vi "Host_SaveToFile.vi"() -> ()   [LabVIEW 2017]
doc: "Dialogue window shows user input for file name.\nSaves all data taken to a file in Data folder.\nIf the explore button is pressed instead, the file explorer wiill be openend and will save data to the specified location."
uses:
  <vilib>/Utility/file.llb/Write Delimited Spreadsheet (string).vi
  Globals/Host_DATAALL.vi
panel:
  in  "Flush Data":bool
  in  "Custom Path":bool
  in  "cancel":bool
  in  "OK Button":bool
  in  "File name":string caption="Enter File Name:"
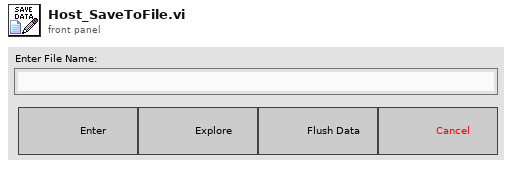
[diagram p1: front panel]
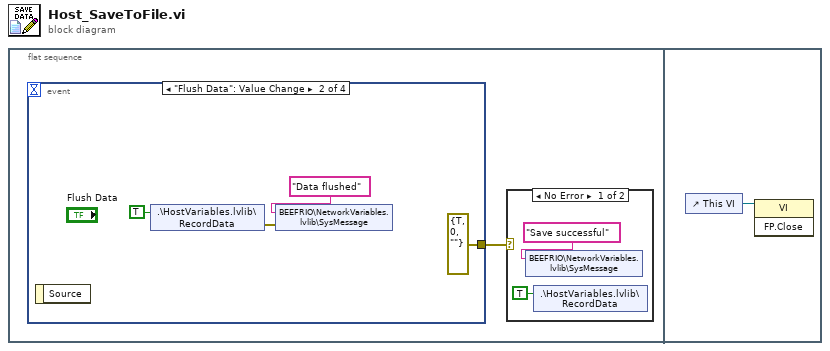
[diagram p0: block diagram]
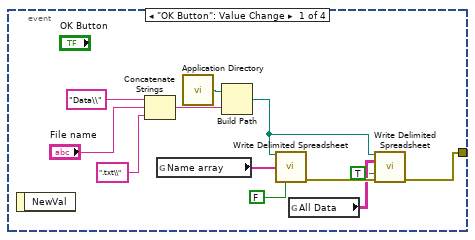
[diagram p3: hidden frame]
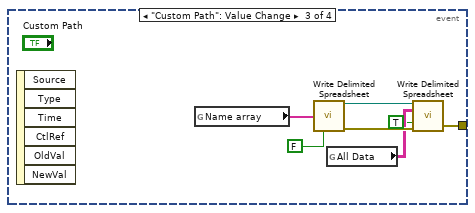
[diagram p4: hidden frame]
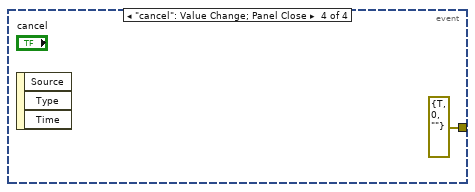
[diagram p5: hidden frame]
diagram:
  n1 = flat-sequence {
    frame #0 {
      n2 = event shown="[1] \"Flush Data\": Value Change" {
        selector: _ -> [_ _ _ _]
        dyn-events: _ -> [_ _ _ _]
        timeout: _ -> [_ _ _ _]
        tunnel: [w4 errorcluster {"status"=TRUE, "code"=0, "source"=""} ("error out") w20 errorcluster {"status"=TRUE, "code"=0, "source"=""} ("error out")] -> w1
        event "OK Button": Value Change {
          n3 = event-data() -> ()  [unwired: 1 in, 1 out]
          n4 = Concatenate Strings("Data\\" ("string"), "File name", ".txt\\" ("string")) -> (w13:string)
          n5 = global read "Host_DATAALL.vi" "Name array"() -> (w9:string[])
          n6 = call <vilib>:"Application Directory.vi"() -> ("Application Directory"=w14:path)
          n7 = Build Path(base path=w14, name or relative path=w13) -> (appended path=w8:path)
          n8 = call-poly <vilib>:"Write Delimited Spreadsheet.vi"("file path (dialog if empty)"=w8, "1D data"=w9, "transpose? (no:F)"=FALSE) -> ("error out"=w7:errorcluster)  [unwired: 11 in, 1 out]
          n9 = global read "Host_DATAALL.vi" "All Data"() -> (w6:string[][])
          n10 = call-poly <vilib>:"Write Delimited Spreadsheet.vi"("file path (dialog if empty)"=w8, "2D data"=w6, "append to file? (new file:F)"=TRUE, "error in (no error)"=w7) -> ("error out"=w4:errorcluster)  [unwired: 10 in, 1 out]
        }
        event "Flush Data": Value Change {
          n11 = event-data() -> ()  [unwired: 1 in, 1 out]
          n12 = shared-variable ".\\HostVariables.lvlib\\RecordData"(TRUE ("RecordData")) -> (error out=w16:errorcluster)  [unwired: 1 in]
          n13 = shared-variable "BEEFRIO\\NetworkVariables.lvlib\\SysMessage"("Data flushed" ("SysMessage"), error in=w16) -> ()  [unwired: 1 out]
        }
        event "Custom Path": Value Change {
          n14 = event-data() -> ()  [unwired: 1 in, 6 out]
          n15 = global read "Host_DATAALL.vi" "Name array"() -> (w25:string[])
          n16 = call-poly <vilib>:"Write Delimited Spreadsheet.vi"("1D data"=w25, "transpose? (no:F)"=FALSE) -> ("new file path (Not A Path if cancelled)"=w21:path, "error out"=w24:errorcluster)  [unwired: 12 in]
          n17 = global read "Host_DATAALL.vi" "All Data"() -> (w23:string[][])
          n18 = call-poly <vilib>:"Write Delimited Spreadsheet.vi"("file path (dialog if empty)"=w21, "2D data"=w23, "append to file? (new file:F)"=TRUE, "error in (no error)"=w24) -> ("error out"=w20:errorcluster)  [unwired: 10 in, 1 out]
        }
        event "cancel": Value Change; Panel Close {
          n19 = event-data() -> ()  [unwired: 1 in, 3 out]
        }
      }
      n20 = case shown="No Error" w1 {
        frame No Error {
          n21 = shared-variable "BEEFRIO\\NetworkVariables.lvlib\\SysMessage"("Save successful" ("SysMessage")) -> ()  [unwired: 1 in, 1 out]
          n22 = shared-variable ".\\HostVariables.lvlib\\RecordData"(TRUE ("RecordData")) -> ()  [unwired: 1 in, 1 out]
        }
        frame Error {
        }
      }
    }
    frame #1 {
      n23 = control-ref of="This VI"() -> (w28:refnum<vi>)
      n24 = invoke class="VI" method="FP.Close"(reference=w28) -> ()  [unwired: 2 in, 3 out]
    }
  }
